vi "Find Tests.vi"(8 "error in (no error)":errorcluster, 10 "Project or Class Path":path, 11 "Execution UI In":refnum<class "Execution UI V2.lvclass">) -> (0 "error out":errorcluster, 3 "Execution UI Out":refnum<class "Execution UI V2.lvclass">)   [LabVIEW 2020, in "Execution UI V2.lvclass"]
uses:
  Execution UI V2.lvclass
  Execution UI V2.lvclass/Execution UI V2.ctl
  LUnit Test Suite/LUnit Test Suite V2.lvclass
  C:/Git/astemes-lunit/source/Rewrite Project/Run/Runnable.lvclass
  Application Framework/Support/Support Utilities/Support Utilities.lvlib
  Test Finder/Test Finder V2.lvclass
  Result Model/Result Model.lvclass
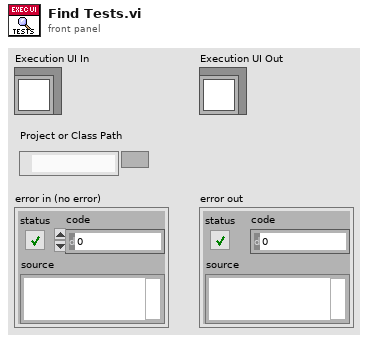
[diagram p1: front panel]
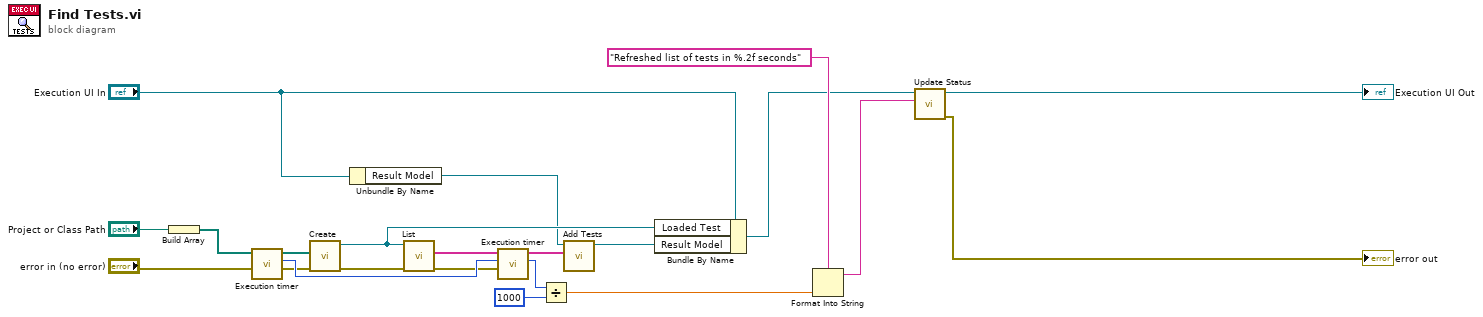
[diagram p0: block diagram]
diagram:
  n1 = Build Array("Project or Class Path") -> (w10:path[])
  n2 = call "Execution timer.vi"("error in (no error)"="error in (no error)") -> ("error out"=w13:errorcluster, "Current or Duration [ms]"=w20:u32)  [unwired: 9 in]
  n3 = call "Create.vi"("error in (no error)"=w13, "File Paths"=w10) -> ("error out"=w12:errorcluster, "LUnit Test Suite V2.lvclass"=w7:refnum<class "LUnit Test Suite V2.lvclass">)  [unwired: 8 in]
  n4 = Unbundle By Name("Execution UI In") -> ("Result Model"=w1:refnum<class "Result Model.lvclass">)
  n5 = call-dynamic "List.vi"("error in (no error)"=w12, "LUnit Test Suite V2 in"=w7) -> ("error out"=w8:errorcluster, "List of Runnables"=w4:string[])  [unwired: 8 in]
  n6 = call "Execution timer.vi"("error in (no error)"=w8, "millisecond timer value"=w20) -> ("Current or Duration [ms]"=w18:u32)  [unwired: 8 in, 1 out]
  n7 = Divide(x=w18, y=u32 1000) -> (x/y=w19:dbl)
  n8 = call "Add Tests.vi"("Tests"=w4, "Result Model In"=w1) -> ("Result Model Out"=w2:refnum<class "Result Model.lvclass">)  [unwired: 9 in]
  n9 = Bundle By Name(cluster="Execution UI In", "Loaded Test"=w7, "Result Model"=w2) -> (w9:refnum<class "Execution UI V2.lvclass">)
  n10 = Format Into String(format string="Refreshed list of tests in %.2f seconds" ("Status"), w19) -> (resulting string=w15:string)  [unwired: 2 in, 1 out]
  n11 = call "Update Status.vi"("Status"=w15, "Execution UI In"=w9) -> ("error out"=→"error out":errorcluster, "Execution UI Out"=→"Execution UI Out":refnum<class "Execution UI V2.lvclass">)  [unwired: 8 in]
